vi "EPICS control.vi"   [LabVIEW 2018]
uses:
  EPICS commands.ctl
  Motor Commands.ctl
types:
  T1 = typedef "Motor Commands.ctl" = enum16{"Get Position", "MoveTo", "MoveToNoWait"}
  T2 = typedef "EPICS commands.ctl" = enum16{"Read Position", "Start Move"}
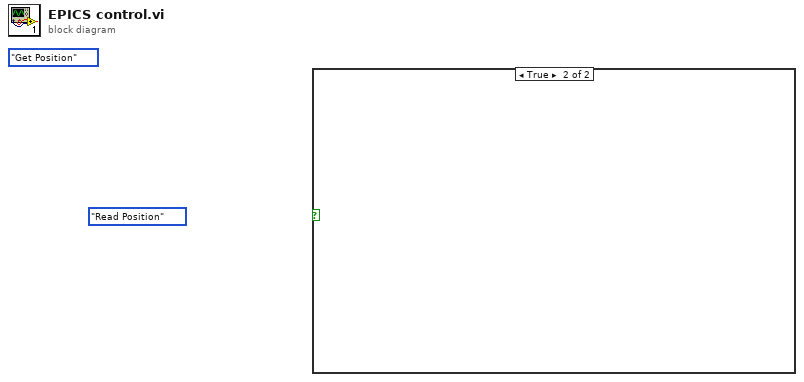
[diagram p0: block diagram]
diagram:
  (unwired) Motor_Commands."Get Position"
  (unwired) EPICS_commands."Read Position"
  n1 = case shown="True" {
    selector: _ -> [_ _]
    frame False {
    }
    frame True {
    }
  }
